vi "Error list.vi"(4 "New Alarm?":bool, 6 "Vehicle":string, 7 "Error array in":string[][](array[string]), 8 "SMS Recipients":u32, 9 "Send SMS":bool, 10 "Error code":dbl, 11 "Counter In":i32=4) -> (0 "Hard alarm?":bool, 2 "Counter Out":i32=4, 3 "Error array out":string[][](array[string]))   [LabVIEW 2014]
uses:
  <vilib>/Utility/file.llb/Write To Spreadsheet File (string).vi
panel:
  out "Boolean array":bool[](array[boolean])
  # "SMS Settings"
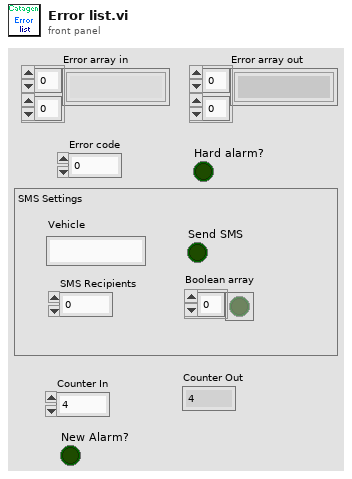
[diagram p1: front panel]
types:
  T1 = cluster{"String":string, "Type":bool, "SMS?":bool}[]
  T2 = cluster{"String":string, "Type":bool, "SMS?":bool}
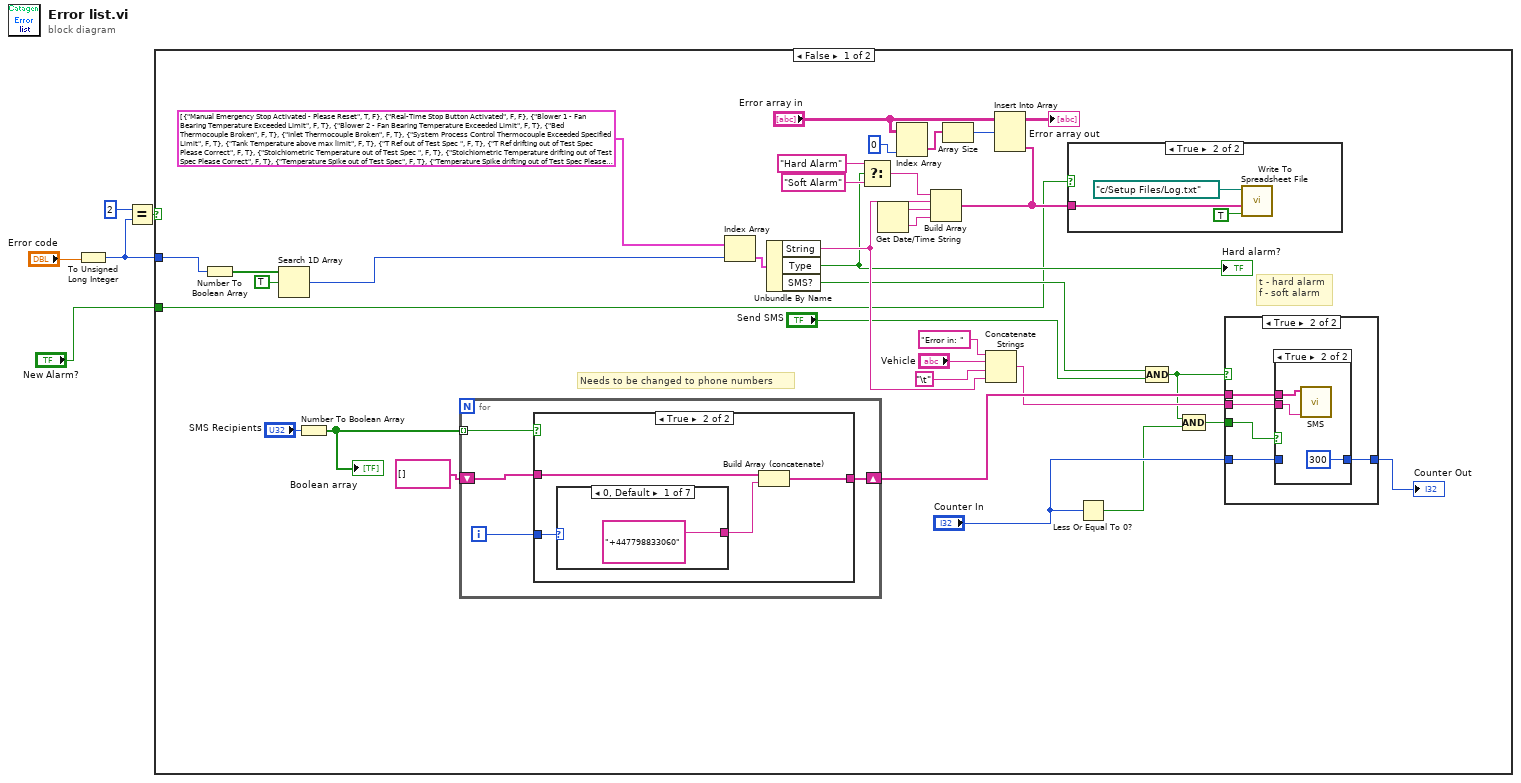
[diagram p0: block diagram]
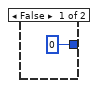
[diagram p3: hidden frame]
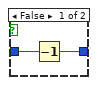
[diagram p4: hidden frame]
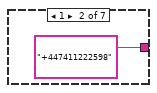
[diagram p6: hidden frame]
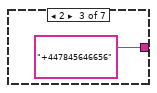
[diagram p7: hidden frame]
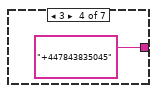
[diagram p8: hidden frame]
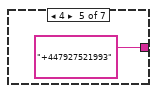
[diagram p9: hidden frame]
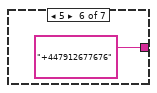
[diagram p10: hidden frame]
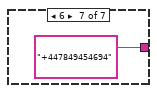
[diagram p11: hidden frame]
diagram:
  n1 = To Unsigned Long Integer(number="Error code") -> (unsigned 32bit integer=w2:u32)
  n2 = Equal?(x=2, y=w2) -> (x = y?=w4:bool)
  n3 = case shown="False" w4 {
    tunnel: w2 -> [w8 _]
    tunnel: "New Alarm?" -> [w6 _]
    frame False {
      # "Needs to be changed to phone numbers"
      # "t - hard alarm\nf - soft alarm"
      n4 = Number To Boolean Array(number=w8) -> (Boolean array=w10:bool[])
      n5 = Search 1D Array(1D array=w10, element=TRUE) -> (index of element=w7:i32)  [unwired: 1 in]
      n6 = Number To Boolean Array(number="SMS Recipients") -> (Boolean array=w27:bool[])
      "Boolean array" <- w27
      n7 = for {
        tunnel: w27 -> [w58] mode=indexing
        shift-right: [w55] -> w25
        shift-left: string[] [] -> [w56]
        i -> [w57]
        n8 = case shown="True" w58 {
          tunnel: w57 -> [_ w63]
          tunnel: w56 -> [w59 w62]
          tunnel: [w59 w60] -> w55
          frame False {
          }
          frame True {
            n9 = case shown="0, Default" w63 {
              tunnel: ["+447798833060" ("String") "+447411222598" ("String") "+447845646656" ("String") "+447843835045" ("String") "+447927521993" ("String") "+447912677676" ("String") "+447849454694" ("String")] -> w61
              frame 0, Default {
              }
              frame 1 {
              }
              frame 2 {
              }
              frame 3 {
              }
              frame 4 {
              }
              frame 5 {
              }
              frame 6 {
              }
            }
            n10 = Build Array (concatenate)(w62, w61) -> (w60:string[])
          }
        }
      }
      n11 = Index Array(array=T1 [{"String"="Manual Emergency Stop Activated - Please Reset", "Type"=TRUE, "SMS?"=FALSE}, {"String"="Real-Time Stop Button Activated", "Type"=FALSE, "SMS?"=FALSE}, {"String"="Blower 1 - Fan Bearing Temperature Exceeded Limit", "Type"=FALSE, "SMS?"=TRUE}, {"String"="Blower 2 - Fan Bearing Temperature Exceeded Limit", "Type"=FALSE, "SMS?"=TRUE}, {"String"="Bed Thermocouple Broken", "Type"=FALSE, "SMS?"=TRUE}, {"String"="Inlet Thermocouple Broken", "Type"=FALSE, "SMS?"=TRUE}, {"String"="System Process Control Thermocouple Exceeded Specified Limit", "Type"=FALSE, "SMS?"=TRUE}, {"String"="Tank Temperature above max limit", "Type"=FALSE, "SMS?"=TRUE}, {"String"="T Ref out of Test Spec ", "Type"=FALSE, "SMS?"=TRUE}, {"String"="T Ref drifting out of Test Spec Please Correct", "Type"=FALSE, "SMS?"=TRUE}, {"String"="Stoichiometric Temperature out of Test Spec ", "Type"=FALSE, "SMS?"=TRUE}, {"String"="Stoichiometric Temperature drifting out of Test Spec Please Correct", "Type"=FALSE, "SMS?"=TRUE}, {"String"="Temperature Spike out of Test Spec", "Type"=FALSE, "SMS?"=TRUE}, {"String"="Temperature Spike drifting out of Test Spec Please Correct", "Type"=FALSE, "SMS?"=TRUE}, {"String"="Control Lambda out of Test Spec", "Type"=FALSE, "SMS?"=TRUE}, {"String"="Control Lambda drifting out of Test Spec Please Correct", "Type"=FALSE, "SMS?"=TRUE}, {"String"="System outside of Pressure range", "Type"=FALSE, "SMS?"=TRUE}, {"String"="Furnace Lambda outside of specified range", "Type"=FALSE, "SMS?"=TRUE}, {"String"="Flow measurement outside of specified range", "Type"=FALSE, "SMS?"=TRUE}, {"String"="", "Type"=FALSE, "SMS?"=FALSE}, {"String"="", "Type"=FALSE, "SMS?"=FALSE}], index=w7) -> (element=w29:T2)
      n12 = Unbundle By Name(w29) -> ("String"=w21:string, "Type"=w18:bool, "SMS?"=w19:bool)
      "Hard alarm?" <- w18
      n13 = Select(t="Hard Alarm", s=w18, f="Soft Alarm") -> (s? t:f=w40:string)
      n14 = Get Date/Time String() -> (date string=w38:string, time string=w39:string)  [unwired: 3 in]
      n15 = Index Array(array="Error array in", index (col)=0 ("index (row)")) -> (element=w34:string[])  [unwired: 1 in]
      n16 = Build Array(w40, w21, w38, w39) -> (w33:string[])
      n17 = Array Size(array=w34) -> (size(s)=w37:i32)
      n18 = Concatenate Strings("Error in: ", "Vehicle", "\t", w21) -> (w20:string)
      n19 = Insert Into Array(array="Error array in", index (row)=w37, new element=w33) -> (→"Error array out":string[][])  [unwired: 1 in]
      n20 = case shown="True" w6 {
        tunnel: w33 -> [_ w41]
        frame False {
        }
        frame True {
          n21 = call-poly <vilib>:"Write To Spreadsheet File.vi"("append to file? (new file:F)"=TRUE, "1D data"=w41, "file path (dialog if empty)"=path "c:/Setup Files/Log.txt") -> ()  [unwired: 5 in, 1 out]
        }
      }
      n22 = Less Or Equal To 0?(x="Counter In") -> (x <= 0?=w14:bool)
      n23 = Compound Arithmetic op=AND(w19, "Send SMS") -> (w13:bool)
      n24 = Compound Arithmetic op=AND(w13, w14) -> (w12:bool)
      n25 = case shown="True" w13 {
        tunnel: w25 -> [_ w49]
        tunnel: w20 -> [_ w48]
        tunnel: "Counter In" -> [_ w47]
        tunnel: [0 w46] -> w11
        tunnel: w12 -> [_ w45]
        frame False {
        }
        frame True {
          n26 = case shown="True" w45 {
            tunnel: w49 -> [_ w53]
            tunnel: w48 -> [_ w52]
            tunnel: w47 -> [w51 _]
            tunnel: [w50 300] -> w46
            frame False {
              n27 = Decrement(x=w51) -> (x-1=w50:i32)
            }
            frame True {
              n28 = call "SMS.vi"("text"=w52, "phoneNumbers"=w53) -> ()  [unwired: 10 in]
            }
          }
        }
      }
      "Counter Out" <- w11
    }
    frame True {
    }
  }
